vi "temp.vi"() -> ()   [LabVIEW 2015]
panel:
  out "x+y":dbl
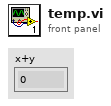
[diagram p1: front panel]
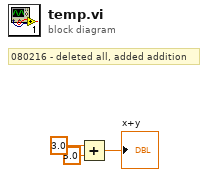
[diagram p0: block diagram]
diagram:
  # "080216 - deleted all, added addition"
  n1 = Add(x=3.0, y=5.0) -> (x+y=→"x+y":dbl)
